vi "Test.vi"() -> ()   [LabVIEW 2011, in "Messenging.lvlib" / "Metronome.lvclass"]
uses:
  Metronome.lvclass
  Interprocess Messenger/Send/Send.lvclass
  Interprocess Messenger/TextVarientMessage/MSG.lvclass
  Interprocess Messenger/Send/Query (static).vi
  Interprocess Messenger/Send/Query (varients).vi
  Interprocess Messenger/EventMessenger/EventMessenger.lvclass
  Interprocess Messenger/VarMessage/Extract Varient (static).vi
  Interprocess Messenger/TextVarientMessage/Write VarMessage.vi
  Interprocess Messenger/VarMessage/VarMessage.lvclass
panel:
  in  "stop":bool
  out "Varient":variant
  out "Label":string
  in  "Period":i32=-1
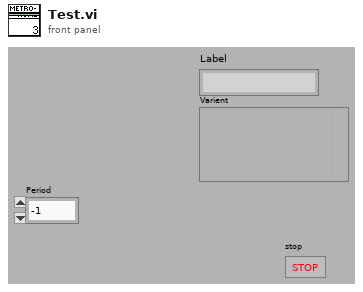
[diagram p1: front panel]
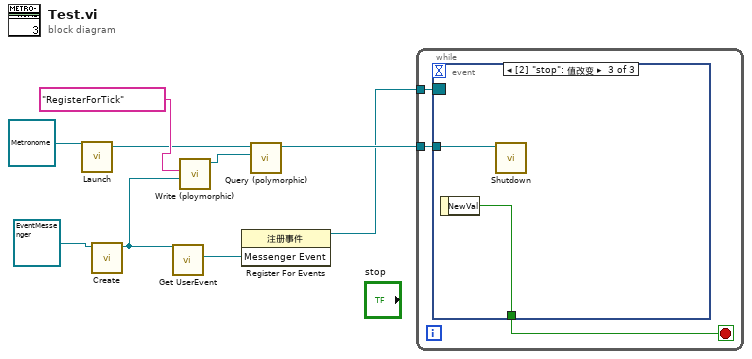
[diagram p0: block diagram]
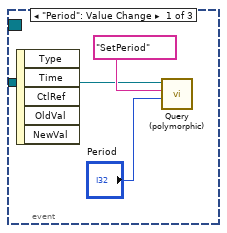
[diagram p2: hidden frame]
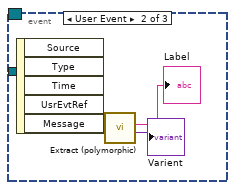
[diagram p3: hidden frame]
diagram:
  n1 = call-dynamic "Launch.vi"("Parallel Process in"=refnum<class "Metronome.lvclass"> refnum ("Parallel Process.lvlib:Metronome.lvclass")) -> ("Parallel Process out"=w7:refnum<class "Metronome.lvclass">)  [unwired: 3 in, 7 out]
  n2 = call-dynamic "Create.vi"("EventMessenger in"=refnum<class "EventMessenger.lvclass"> refnum ("Messenging.lvlib:Event Messenger")) -> ("EventMessenger out"=w3:refnum<class "EventMessenger.lvclass">)  [unwired: 1 in, 9 out]
  n3 = call-dynamic "Get UserEvent.vi"("EventMessenger"=w3) -> ("Messenger Event"=w2:refnum<user-event>)  [unwired: 1 in, 9 out]
  n4 = call-poly "Write (ploymorphic).vi"("Varient"=w3, "Label"="RegisterForTick") -> ("Message"=w6:refnum<class "VarMessage.lvclass">)  [unwired: 1 in, 8 out]
  n5 = register-events(w2) -> (reference out=w1:refnum<event-registration>)  [unwired: 2 in, 1 out]
  n6 = call-poly "Query (polymorphic).vi"("Message"=w6, "MSR Parent"=w7) -> ("MSR Parent"=w5:refnum<class "Metronome.lvclass">)  [unwired: 2 in, 7 out]
  n7 = while {
    tunnel: w5 -> [w12]
    tunnel: w1 -> [w11]
    stop <- w10 stop-if-true
    n8 = event shown="[2] \"stop\": 值改变" {
      selector: w11 -> [_ _ _]
      dyn-events: _ -> [_ _ _]
      timeout: _ -> [_ _ _]
      tunnel: w12 -> [w14 _ w19]
      tunnel: [_ _ w20] -> w10
      event "Period": Value Change {
        n9 = event-data() -> ()  [unwired: 6 out]
        n10 = call-poly "Query (polymorphic).vi"("Varient"="Period", "Label"="SetPeriod", "MSR Parent"=w14) -> ()  [unwired: 2 in, 7 out]
      }
      event User Event {
        n11 = event-data() -> ("Message"=w18:refnum<class "MSG.lvclass">)  [unwired: 5 out]
        n12 = call-poly "Extract (polymorphic).vi"("Interprocess Message in"=w18) -> ("Varient"=→"Varient":variant, "Label"=→"Label":string)  [unwired: 1 in, 8 out]
      }
      event "stop": Value Change {
        n13 = event-data() -> ("NewVal"=w20:bool)  [unwired: 1 out]
        n14 = call-dynamic "Shutdown.vi"("Parallel Process in"=w19) -> ()  [unwired: 3 in, 8 out]
      }
    }
  }
